vi "Test Live Data Scaling.vi"() -> ()   [LabVIEW 2016]
uses:
  Frames & Messages/TypeDefs/Message Config.ctl
  Frames & Messages/TypeDefs/Command Config.ctl
  Frames & Messages/TypeDefs/Message Control.ctl
  Bus Controller/TypeDefs/Bus Controller Configuration.ctl
  Remote Terminal/TypeDefs/RT Configuration.ctl
  Remote Terminal/TypeDefs/Command Configuration.ctl
  Remote Terminal/TypeDefs/Command Type.ctl
  1553 SubComponent/TypeDefs/Parameter Table Data.ctl
  1553 SubComponent/TypeDefs/Scaling Information.ctl
  Remote Terminal/Remote Terminal.lvclass
  D:/SVN/Products/BCI-1553/Software/Development/2016/RealTime/1553 SubComponent/1553 SubComponent.lvclass
  Bus Controller/Bus Controller.lvclass
  Frames & Messages/Major Frame/Major Frame.lvclass
  1553 Board/1553 Board.lvclass
  Frames & Messages/Message/Message.lvclass
  BCI-1553 API.lvlib
  1553 SubComponent/1553 SubComponent.lvclass
  Frames & Messages/Minor Frame/Minor Frame.lvclass
  1553 Component/1553 Component.lvclass
  Utilities/FPGA Interface/FPGA Interface.lvclass
panel:
  out "Scaled Data":dbl[][](array[numeric])
  out "Parameters":string[][](array[string])
  in  "stop":bool
  in  "New Value":dbl format="%#.6g"
  in  "Parameter to Update":string
  in  "Component Index":i32
  in  "Write Scaled Data":bool
  in  "Read Scaled Data":bool
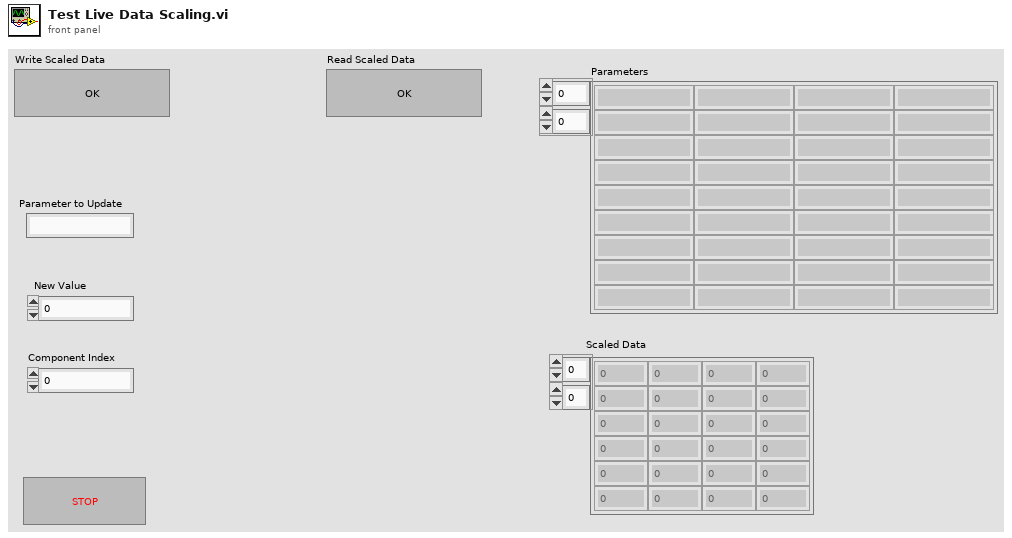
[diagram p1: front panel]
types:
  T1 = typedef "BCI-1553 API.lvlib/1553 SubComponent.lvclass/Scaling Information.ctl" = cluster{"Bit Offset":i32, "Bit Count":i32, "LSB Resolution":dbl, "2's Complement":bool, "Big Endian":bool, "Sign Bit":bool}
  T2 = typedef "BCI-1553 API.lvlib/1553 SubComponent.lvclass/Parameter Table Data.ctl" = cluster{"Parameter Name":string, "Base Word":u16, "Address":u16, "Value":u64, "Mask":u16[], "Scaling Info":T1}
  T3 = typedef "BCI-1553 API.lvlib/Remote Terminal.lvclass/Command Configuration.ctl" = cluster{"Command Type":T4, "Mode Code ID (1-32)":u16, "SubAddress (1-30)":u16, "Word Count (1-32)":u16, "Illegal Command":bool, "Broadcast":bool, "Data":u16[], "Data Fields":T2[]}
  T4 = typedef "BCI-1553 API.lvlib/Remote Terminal.lvclass/Command Type.ctl" = enum16{"Transmit", "Receive", "Mode Code Tx", "Mode Code Rx"}
  T5 = typedef "BCI-1553 API.lvlib/Remote Terminal.lvclass/RT Configuration.ctl" = cluster{"RT-RT TimeOut (us)":u8, "Inhibit Bus A":bool, "Inhibit Bus B":bool, "Broadcast CMD Invalid":bool, "UnDef MCs Invalid":bool, "Notice 2 Data Storage":bool, "SMCP":bool, "Temp RX Buffer":bool, "Alt BIT Enable":bool, "Auto Bus Shutdown":bool, "MC 17 Sync":u8, "MC 16 SR Reset":bool, "MC 8 Reset":bool}
  T6 = typedef "BCI-1553 API.lvlib/Bus Controller.lvclass/Bus Controller Configuration.ctl" = cluster{"BC Timeout":u16, "BC Retry":bool, "BC Second Retry":bool, "BC Retry Alt Bus":bool, "BC Second Retry Alt Bus":bool, "BC Retry on Status Bit":bool, "Msg Error No Data Valid":bool, "Busy Status No Data Valid":bool, "Msg Gap Timer":bool, "Watchdog Timer":bool, "Time Tag Sync":bool, "Even Time Tag Sync":bool, "Gap Check":bool, "Broadcast Mask Enable":bool}
  T7 = typedef "BCI-1553 API.lvlib/Message Config.ctl" = cluster{"Time to Next Msg (4 us)":u16, "Command Config":T8, "Message Control":T9}
  T8 = typedef "BCI-1553 API.lvlib/Command Config.ctl" = cluster{"Command Type":enum16{"Transmit", "Receive"}, "Terminal Address (0-30)":u16, "SubAddress (1-30)":u16, "WC/MC (1-32)":u16, "Command Data":u16[]}
  T9 = typedef "BCI-1553 API.lvlib/Message Control.ctl" = cluster{"MC17 Time Sync":bool, "Error Mask":bool, "Service Request Mask":bool, "Busy Mask":bool, "SubSystem Flag Mask":bool, "Terminal Flag Mask":bool, "Reserved Mask":bool, "Retry":bool, "Bus A / !Bus B":bool, "Self-Test Loopback":bool, "Broadcast Mask":bool, "EoM Interrupt":bool, "Mode Code Format":bool, "Broadcast Format":bool, "RT-RT Format":bool}
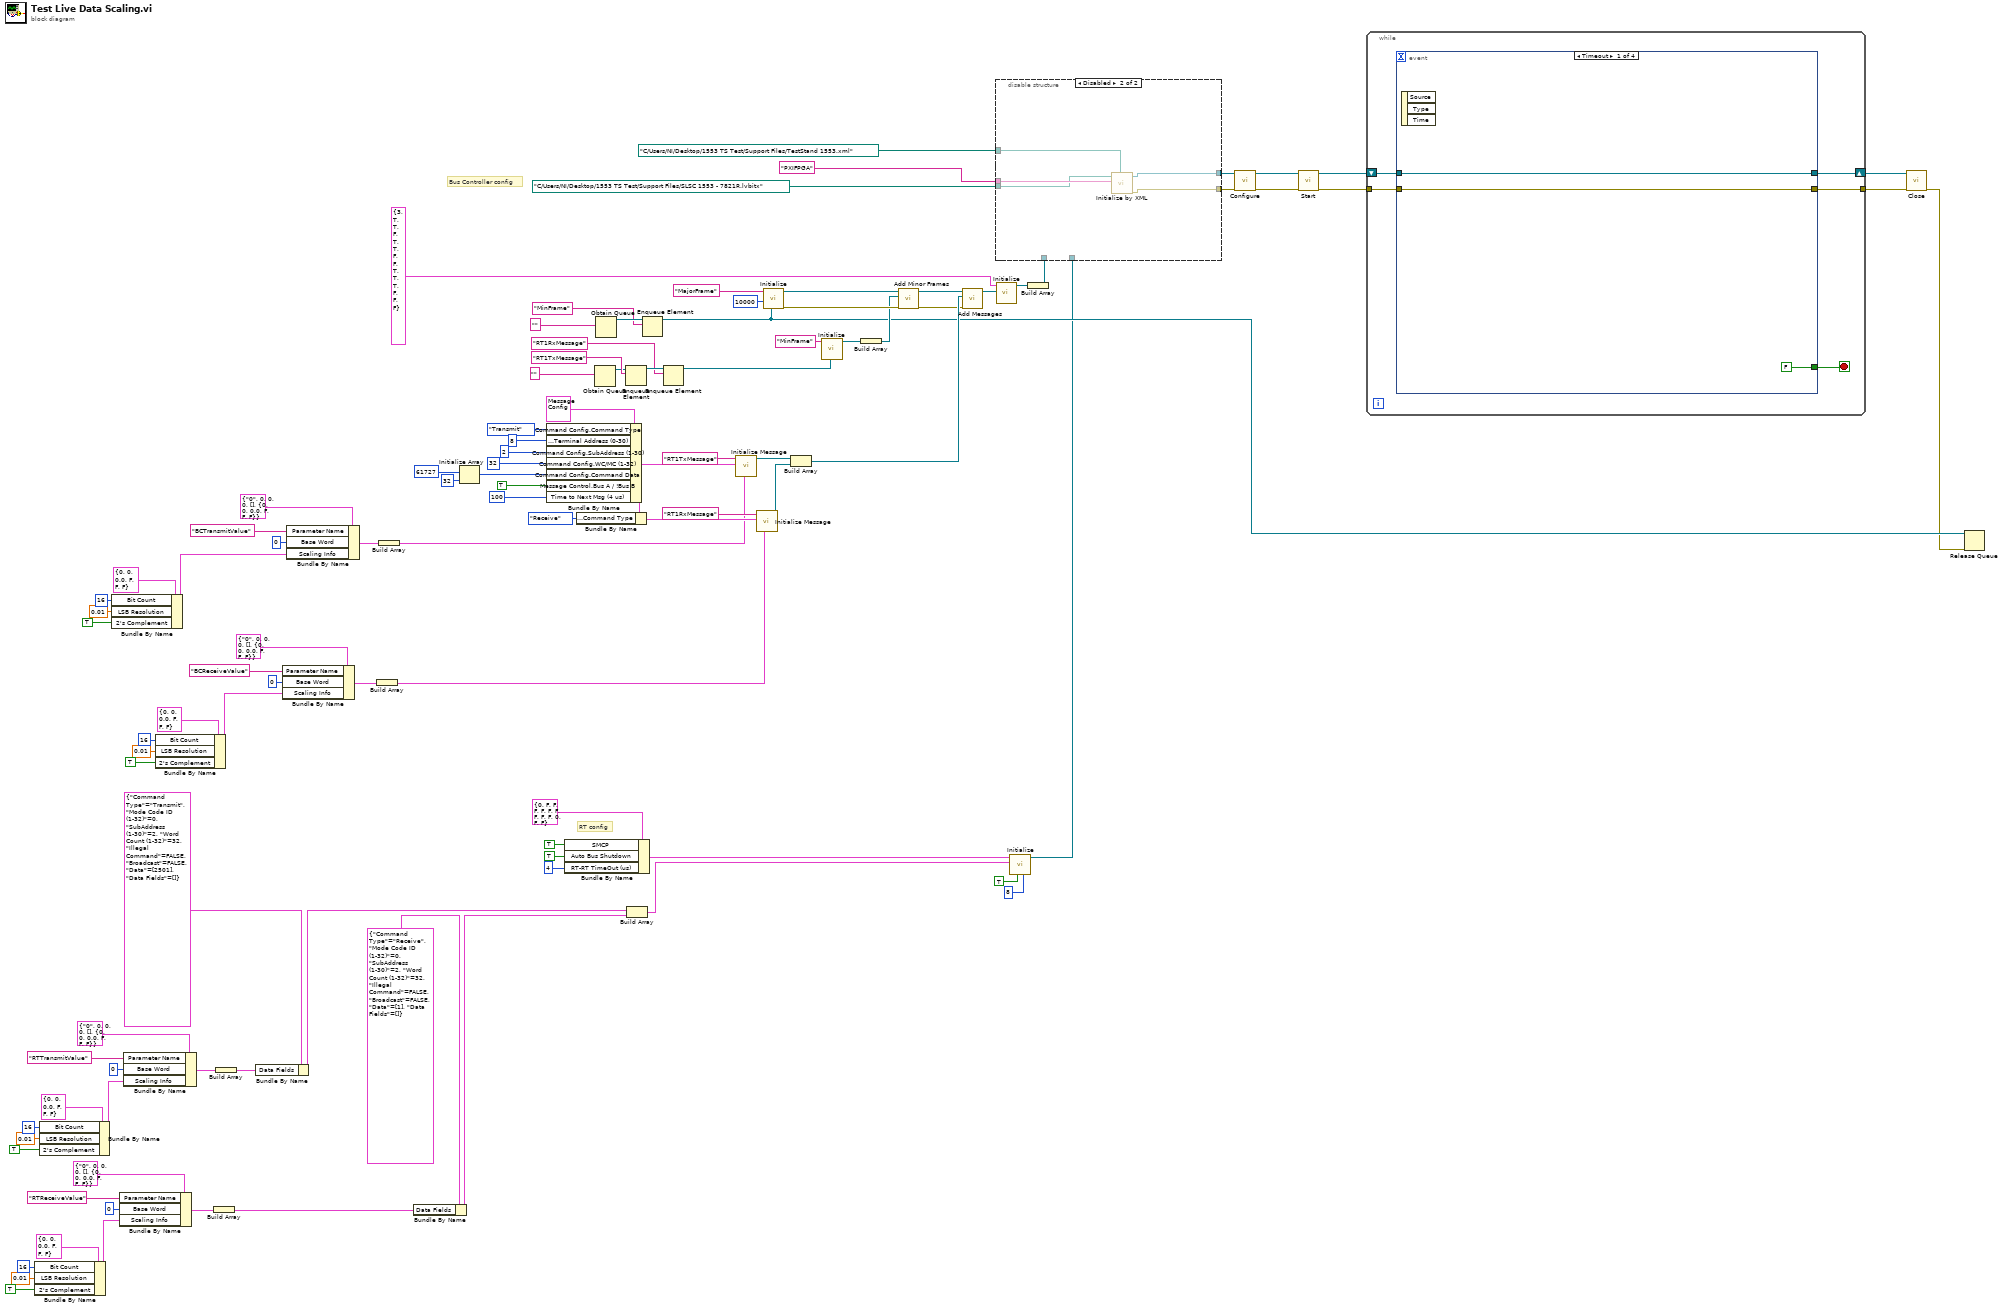
[diagram p0: block diagram]
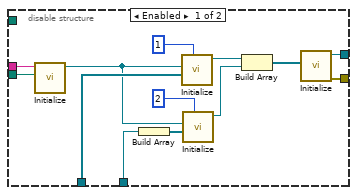
[diagram p2: hidden frame]
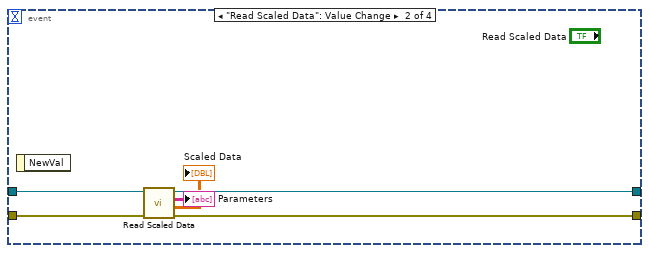
[diagram p3: hidden frame]
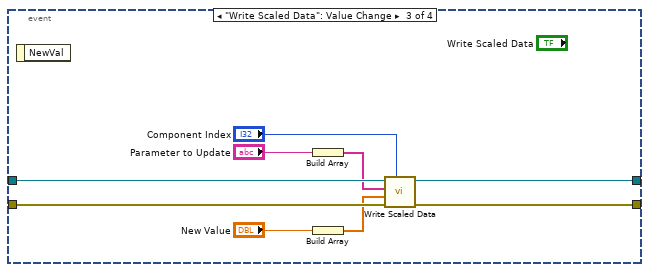
[diagram p4: hidden frame]
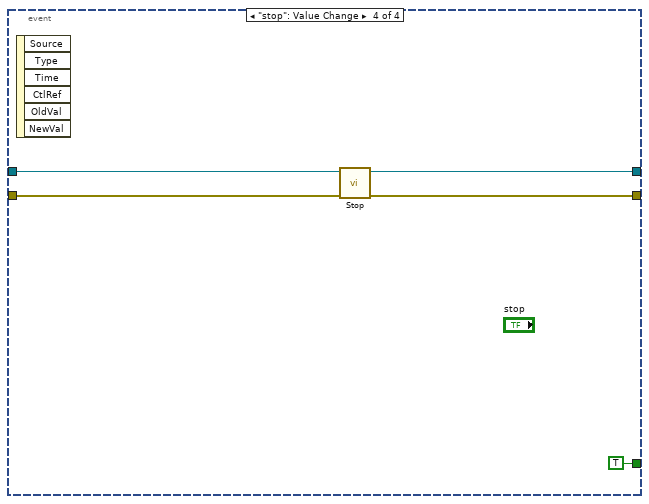
[diagram p5: hidden frame]
diagram:
  # "RT config"
  # "Bus Controller config"
  n1 = Bundle By Name(cluster=T1 {"Bit Offset"=0, "Bit Count"=0, "LSB Resolution"=0.0, "2's Complement"=FALSE, "Big Endian"=FALSE, "Sign Bit"=FALSE} ("Scaling Info"), "Bit Count"=16, "LSB Resolution"=0.01, "2's Complement"=TRUE) -> (w23:T1)
  n2 = Bundle By Name(cluster=T1 {"Bit Offset"=0, "Bit Count"=0, "LSB Resolution"=0.0, "2's Complement"=FALSE, "Big Endian"=FALSE, "Sign Bit"=FALSE} ("Scaling Info"), "Bit Count"=16, "LSB Resolution"=0.01, "2's Complement"=TRUE) -> (w15:T1)
  n3 = Bundle By Name(cluster=T1 {"Bit Offset"=0, "Bit Count"=0, "LSB Resolution"=0.0, "2's Complement"=FALSE, "Big Endian"=FALSE, "Sign Bit"=FALSE} ("Scaling Info"), "Bit Count"=16, "LSB Resolution"=0.01, "2's Complement"=TRUE) -> (w44:T1)
  n4 = Bundle By Name(cluster=T2 {"Parameter Name"="0", "Base Word"=0, "Address"=0, "Value"=0, "Mask"=[], "Scaling Info"={"Bit Offset"=0, "Bit Count"=0, "LSB Resolution"=0.0, "2's Complement"=FALSE, "Big Endian"=FALSE, "Sign Bit"=FALSE}} ("Parameter Table Data"), "Parameter Name"="RTReceiveValue", "Base Word"=u16 0, "Scaling Info"=w23) -> (w28:T2)
  n5 = Bundle By Name(cluster=T2 {"Parameter Name"="0", "Base Word"=0, "Address"=0, "Value"=0, "Mask"=[], "Scaling Info"={"Bit Offset"=0, "Bit Count"=0, "LSB Resolution"=0.0, "2's Complement"=FALSE, "Big Endian"=FALSE, "Sign Bit"=FALSE}} ("Parameter Table Data"), "Parameter Name"="RTTransmitValue", "Base Word"=u16 0, "Scaling Info"=w15) -> (w19:T2)
  n6 = Bundle By Name(cluster=T1 {"Bit Offset"=0, "Bit Count"=0, "LSB Resolution"=0.0, "2's Complement"=FALSE, "Big Endian"=FALSE, "Sign Bit"=FALSE} ("Scaling Info"), "Bit Count"=16, "LSB Resolution"=0.01, "2's Complement"=TRUE) -> (w35:T1)
  n7 = Build Array(w28) -> (w7:T2[])
  n8 = Build Array(w19) -> (w10:T2[])
  n9 = Bundle By Name(cluster=T3 {"Command Type"=enum."Transmit", "Mode Code ID (1-32)"=0, "SubAddress (1-30)"=2, "Word Count (1-32)"=32, "Illegal Command"=FALSE, "Broadcast"=FALSE, "Data"=[2501], "Data Fields"=[]} ("CMD Configuration"), "Data Fields"=w10) -> (w8:T3)
  n10 = Bundle By Name(cluster=T2 {"Parameter Name"="0", "Base Word"=0, "Address"=0, "Value"=0, "Mask"=[], "Scaling Info"={"Bit Offset"=0, "Bit Count"=0, "LSB Resolution"=0.0, "2's Complement"=FALSE, "Big Endian"=FALSE, "Sign Bit"=FALSE}} ("Parameter Table Data"), "Parameter Name"="BCReceiveValue", "Base Word"=u16 0, "Scaling Info"=w35) -> (w30:T2)
  n11 = Bundle By Name(cluster=T2 {"Parameter Name"="0", "Base Word"=0, "Address"=0, "Value"=0, "Mask"=[], "Scaling Info"={"Bit Offset"=0, "Bit Count"=0, "LSB Resolution"=0.0, "2's Complement"=FALSE, "Big Endian"=FALSE, "Sign Bit"=FALSE}} ("Parameter Table Data"), "Parameter Name"="BCTransmitValue", "Base Word"=u16 0, "Scaling Info"=w44) -> (w40:T2)
  n12 = Build Array(w30) -> (w29:T2[])
  n13 = Build Array(w40) -> (w39:T2[])
  n14 = Bundle By Name(cluster=T3 {"Command Type"=enum."Receive", "Mode Code ID (1-32)"=0, "SubAddress (1-30)"=2, "Word Count (1-32)"=32, "Illegal Command"=FALSE, "Broadcast"=FALSE, "Data"=[1], "Data Fields"=[]} ("CMD Configuration"), "Data Fields"=w7) -> (w5:T3)
  n15 = Initialize Array(u16 61727 ("Data"), 32 ("dimension size")) -> (w56:u16[])
  n16 = Bundle By Name(cluster=T7 {"Time to Next Msg (4 us)"=100, "Command Config"={"Command Type"=enum."Transmit", "Terminal Address (0-30)"=0, "SubAddress (1-30)"=0, "WC/MC (1-32)"=0, "Command Data"=[]}, "Message Control"={"MC17 Time Sync"=FALSE, "Error Mask"=FALSE, "Service Request Mask"=FALSE, "Busy Mask"=FALSE, "SubSystem Flag Mask"=FALSE, "Terminal Flag Mask"=FALSE, "Reserved Mask"=FALSE, "Retry"=FALSE, "Bus A / !Bus B"=FALSE, "Self-Test Loopback"=FALSE, "Broadcast Mask"=FALSE, "EoM Interrupt"=FALSE, "Mode Code Format"=FALSE, "Broadcast Format"=FALSE, "RT-RT Format"=FALSE}} ("Message  Config"), "Command Config.Command Type"=enum16{"Transmit", "Receive"}."Transmit", "Command Config.Terminal Address (0-30)"=u16 8, "Command Config.SubAddress (1-30)"=u16 2, "Command Config.WC/MC (1-32)"=u16 32, "Command Config.Command Data"=w56, "Message Control.Bus A / !Bus B"=TRUE, "Time to Next Msg (4 us)"=u16 100) -> (w85:T7)
  n17 = Bundle By Name(cluster=T5 {"RT-RT TimeOut (us)"=0, "Inhibit Bus A"=FALSE, "Inhibit Bus B"=FALSE, "Broadcast CMD Invalid"=FALSE, "UnDef MCs Invalid"=FALSE, "Notice 2 Data Storage"=FALSE, "SMCP"=FALSE, "Temp RX Buffer"=FALSE, "Alt BIT Enable"=FALSE, "Auto Bus Shutdown"=FALSE, "MC 17 Sync"=0, "MC 16 SR Reset"=FALSE, "MC 8 Reset"=FALSE} ("RT Configuration"), "SMCP"=TRUE, "Auto Bus Shutdown"=TRUE ("Inhibit Bus A"), "RT-RT TimeOut (us)"=u8 4) -> (w84:T5)
  n18 = Bundle By Name(cluster=w85, "Command Config.Command Type"=enum16{"Transmit", "Receive"}."Receive") -> (w86:T7)
  n19 = Obtain Queue(element data type="") -> (queue out=w67:refnum<queue>)  [unwired: 4 in, 2 out]
  n20 = Obtain Queue(element data type="") -> (queue out=w79:refnum<queue>)  [unwired: 4 in, 2 out]
  n21 = Enqueue Element(queue=w67, element="RT1TxMessage") -> (queue out=w62:refnum<queue>)  [unwired: 2 in, 2 out]
  n22 = Build Array(w8, w5) -> (w51:T3[])
  n23 = Enqueue Element(queue=w79, element="MinFrame") -> (queue out=w55:refnum<queue>)  [unwired: 2 in, 2 out]
  n24 = Enqueue Element(queue=w62, element="RT1RxMessage") -> (queue out=w49:refnum<queue>)  [unwired: 2 in, 2 out]
  n25 = call "Initialize Message.vi"("Parameters"=w39, "Message  Config"=w85, "ID"="RT1TxMessage") -> ("Message out"=w100:refnum<class "Message.lvclass">)  [unwired: 7 in, 1 out]
  n26 = call "Initialize Message.vi"("Parameters"=w29, "Message  Config"=w86, "ID"="RT1RxMessage") -> ("Message out"=w99:refnum<class "Message.lvclass">)  [unwired: 7 in, 1 out]
  n27 = call "Initialize.vi"("Schedule"=w55, "Minor Frame Time (100 us)"=u16 10000, "ID"="MajorFrame") -> ("error out"=w75:errorcluster, "Major Frame out"=w77:refnum<class "Major Frame.lvclass">)  [unwired: 7 in]
  n28 = Build Array(w100, w99) -> (w80:refnum<class "Message.lvclass">[])
  n29 = call "Initialize.vi"("Schedule"=w49, "ID"="MinFrame") -> ("Minor Frame out"=w73:refnum<class "Minor Frame.lvclass">)  [unwired: 8 in, 1 out]
  n30 = Build Array(w73) -> (w72:refnum<class "Minor Frame.lvclass">[])
  n31 = call-dynamic "Add Minor Frames.vi"("error in (no error)"=w75, "Minor Frames"=w72, "Major Frame in"=w77) -> ("error out"=w74:errorcluster, "Major Frame out"=w76:refnum<class "Major Frame.lvclass">)  [unwired: 7 in]
  n32 = call-dynamic "Add Messages.vi"("error in (no error)"=w74, "Messages"=w80, "Major Frame in"=w76) -> ("Major Frame out"=w81:refnum<class "Major Frame.lvclass">)  [unwired: 7 in, 1 out]
  n33 = call "Initialize.vi"("Major Frame"=w81, "Configuration"=T6 {"BC Timeout"=3, "BC Retry"=TRUE, "BC Second Retry"=TRUE, "BC Retry Alt Bus"=FALSE, "BC Second Retry Alt Bus"=TRUE, "BC Retry on Status Bit"=TRUE, "Msg Error No Data Valid"=FALSE, "Busy Status No Data Valid"=FALSE, "Msg Gap Timer"=TRUE, "Watchdog Timer"=TRUE, "Time Tag Sync"=TRUE, "Even Time Tag Sync"=FALSE, "Gap Check"=FALSE, "Broadcast Mask Enable"=FALSE}) -> ("Bus Controller out"=w104:refnum<class "Bus Controller.lvclass">)  [unwired: 8 in, 1 out]
  n34 = call "Initialize.vi"("RT Address (0-30)"=u8 8, "RT 1?"=TRUE, "Commands"=w51, "RT Configuration"=w84) -> ("Remote Terminal out"=w50:refnum<class "Remote Terminal.lvclass">)  [unwired: 6 in, 1 out]
  n35 = Build Array(w104) -> (w91:refnum<class "Bus Controller.lvclass">[])
  n36 = disable-structure shown="Disabled" {
    disable-tunnel: w91 -> [w113 _]
    disable-tunnel: path "C:/Users/NI/Desktop/1553 TS Test/Support Files/SLSC 1553 - 7821R.lvbitx" ("Bitfile path") -> [w118 w123]
    disable-tunnel: [w116 w121] -> w83
    disable-tunnel: [w115 w120] -> w82
    disable-tunnel: "PXIFPGA" ("Device address") -> [w114 w124]
    disable-tunnel: path "C:/Users/NI/Desktop/1553 TS Test/Support Files/TestStand 1553.xml" ("XML File") -> [_ w122]
    disable-tunnel: w50 -> [w110 _]
    frame Enabled {
      n37 = call "Initialize.vi"("Bitfile path"=w118, "Device address"=w114) -> ("FPGA Interface out"=w111:refnum<class "FPGA Interface.lvclass">)  [unwired: 8 in, 1 out]
      n38 = Build Array(w110) -> (w109:refnum<class "Remote Terminal.lvclass">[])
      n39 = call "Initialize.vi"("Component ID (1-8)"=u8 1, "SubComponents"=w113, "FPGA Interface"=w111) -> ("1553 Component out"=w107:refnum<class "1553 Component.lvclass">)  [unwired: 7 in, 1 out]
      n40 = call "Initialize.vi"("Component ID (1-8)"=u8 2, "SubComponents"=w109, "FPGA Interface"=w111) -> ("1553 Component out"=w108:refnum<class "1553 Component.lvclass">)  [unwired: 7 in, 1 out]
      n41 = Build Array(w107, w108) -> (w117:refnum<class "1553 Component.lvclass">[])
      n42 = call "Initialize.vi"("Components"=w117) -> ("error out"=w115:errorcluster, "1553 Board out"=w116:refnum<class "1553 Board.lvclass">)  [unwired: 9 in]
    }
    frame Disabled {
      n43 = call "Initialize by XML.vi"("XML File"=w122, "FPGA Device Address"=w124, "FPGA Bitfile"=w123) -> ("error out"=w120:errorcluster, "1553 Board out"=w121:refnum<class "1553 Board.lvclass">)  [unwired: 7 in]
    }
  }
  n44 = call-dynamic "Configure.vi"("error in (no error)"=w82, "1553 Board in"=w83) -> ("error out"=w2:errorcluster, "1553 Board out"=w4:refnum<class "1553 Board.lvclass">)  [unwired: 8 in]
  n45 = call-dynamic "Start.vi"("error in (no error)"=w2, "1553 Board in"=w4) -> ("error out"=w1:errorcluster, "1553 Board out"=w3:refnum<class "1553 Board.lvclass">)  [unwired: 8 in]
  n46 = while {
    tunnel: w1 -> [w125]
    shift-right: [w128] -> w54
    shift-left: w3 -> [w127]
    tunnel: [w126] -> w52
    stop <- w129 stop-if-true
    n47 = event shown="[0] Timeout" {
      selector: _ -> [_ _ _ _]
      dyn-events: _ -> [_ _ _ _]
      timeout: _ -> [_ _ _ _]
      tunnel: [FALSE _ _ TRUE] -> w129
      tunnel: [w131 w137 w146 w150] -> w128
      tunnel: w127 -> [w131 w138 w147 w151]
      tunnel: [w130 w135 w145 w148] -> w126
      tunnel: w125 -> [w130 w136 w144 w149]
      event Timeout {
        n48 = event-data() -> ()  [unwired: 1 in, 3 out]
      }
      event "Read Scaled Data": Value Change {
        n49 = event-data() -> ()  [unwired: 1 in, 1 out]
        n50 = call-dynamic "Read Scaled Data.vi"("error in (no error)"=w136, "1553 Board in"=w138) -> ("error out"=w135:errorcluster, "Scaled Data"=→"Scaled Data":dbl[][], "Parameters"=→"Parameters":string[][], "1553 Board out"=w137:refnum<class "1553 Board.lvclass">)  [unwired: 6 in]
      }
      event "Write Scaled Data": Value Change {
        n51 = event-data() -> ()  [unwired: 1 in, 1 out]
        n52 = Build Array("Parameter to Update") -> (w141:string[])
        n53 = Build Array("New Value") -> (w139:dbl[])
        n54 = call-dynamic "Write Scaled Data.vi"("Component Index"="Component Index", "error in (no error)"=w144, "Scaled Data"=w139, "Parameters"=w141, "1553 Board in"=w147) -> ("error out"=w145:errorcluster, "1553 Board out"=w146:refnum<class "1553 Board.lvclass">)  [unwired: 5 in]
      }
      event "stop": Value Change {
        n55 = event-data() -> ()  [unwired: 1 in, 6 out]
        n56 = call-dynamic "Stop.vi"("error in (no error)"=w149, "1553 Board in"=w151) -> ("error out"=w148:errorcluster, "1553 Board out"=w150:refnum<class "1553 Board.lvclass">)  [unwired: 8 in]
      }
    }
  }
  n57 = call-dynamic "Close.vi"("error in (no error)"=w52, "1553 Board in"=w54) -> ("error out"=w53:errorcluster)  [unwired: 9 in]
  n58 = Release Queue(queue=w55, error in (no error)=w53) -> ()  [unwired: 1 in, 3 out]
